vi "Log Event.vi"(6 "Event Time":timestamp, 7 "Event Level":T1, 8 "error in (no error)":errorcluster, 10 "Data To Log":string, 11 "SourceID":string) -> (0 "error out":errorcluster)   [LabVIEW 2019, in "Singleton Event Log.lvlib"]
uses:
  <vilib>/gpm_packages/@cs/event-logger/Source/Composed Log/Singleton Event Log/Singleton Event Log.lvlib
  <vilib>/gpm_packages/@cs/event-logger/Source/Composed Log/Types/Log Level.ctl
  <vilib>/gpm_packages/@cs/event-logger/Source/Composed Log/LoggerReference/LoggerReference.lvclass/LoggerReference.ctl
  <vilib>/gpm_packages/@cs/event-logger/Source/Composed Log/LoggerReference/Log.vi
  <vilib>/gpm_packages/@cs/event-logger/Source/Composed Log/LoggerReference/Get Valid Event Time.vi
  <vilib>/gpm_packages/@cs/event-logger/Source/Composed Log/LoggerReference/Remove Stale Logs.vi
  <vilib>/gpm_packages/@cs/event-logger/Source/Composed Log/LoggerReference/LoggerReference.lvclass
  <vilib>/gpm_packages/@cs/event-logger/Source/Composed Log/Composed Log.lvlib
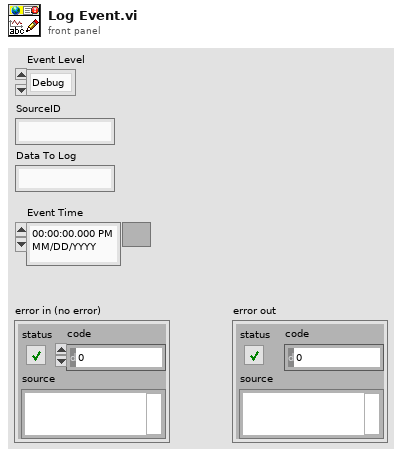
[diagram p1: front panel]
types:
  T1 = typedef "Composed Log.lvlib/Log Level.ctl" = enum16{"Debug", "Info", "Warning", "Error", "Critical"}
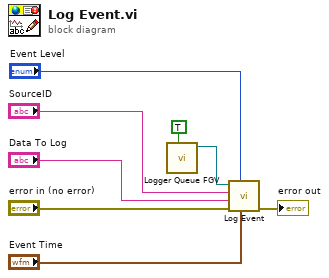
[diagram p0: block diagram]
diagram:
  n1 = call <vilib>:"Logger Queue FGV.vi"("Read?"=TRUE) -> ("LogReference Instance Out"=w2:refnum<class "LoggerReference.lvclass">)  [unwired: 10 in]
  n2 = call <vilib>:"Log Event.vi"("Event Time"="Event Time", "Event Level"="Event Level", "error in (no error)"="error in (no error)", "Data To Log"="Data To Log", "SourceID"="SourceID", "Log Instance"=w2) -> ("error out"=→"error out":errorcluster)  [unwired: 4 in, 1 out]
